vi "Support Globals.vi"() -> ()   [LabVIEW 2021]
panel:
  out "Screen checked?":bool
  out "Close?":bool
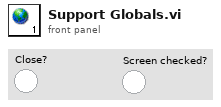
[diagram p1: front panel]
diagram:
